vi "NXT_MIDBRAIN Wait For Buffer To Fill.vi"(4 "Buffer Length":u8, 5 "ModuleName":string, 6 "error in (no error)":errorcluster, 7 "Refnum in":T1) -> (2 "error out":errorcluster, 3 "Refnum out":T1)   [LabVIEW 2012]
uses:
  <vilib>/NXT/NXT Controls/NXTSyscallRefnum.ctl
  <resource>/objmgr/NXTInputOutput.rc
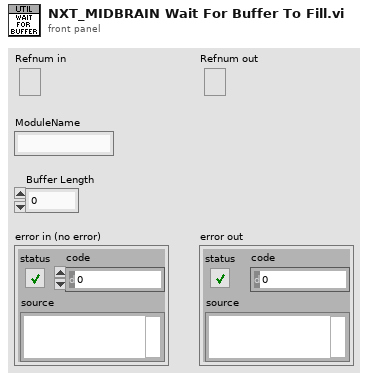
[diagram p1: front panel]
types:
  T1 = typedef "NXTSyscallRefnum.ctl" = refnum<k21>
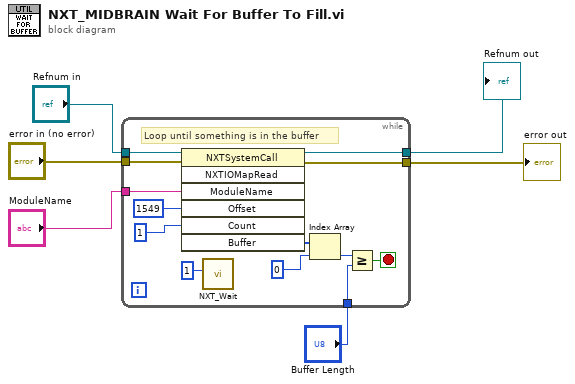
[diagram p0: block diagram]
diagram:
  n1 = while {
    tunnel: [w15] -> w3
    tunnel: [w14] -> w4
    tunnel: "Refnum in" -> [w13]
    tunnel: "error in (no error)" -> [w12]
    tunnel: "ModuleName" -> [w11]
    tunnel: "Buffer Length" -> [w7]
    stop <- w10 stop-if-true
    # "Loop until something is in the buffer"
    n2 = invoke class="NXTSystemCall" method="NXTIOMapRead"(reference=w13, error in=w12, "ModuleName"=w11, "Offset"=u16 1549, "Count"=u16 1) -> (reference out=w15:T1, error out=w14:errorcluster, "Buffer"=w18:u8[])  [unwired: 2 in, 4 out]
    n3 = call <vilib>:"NXT_Wait.vi"("Wait (ms)"=u32 1) -> ()  [unwired: 9 in, 2 out]
    n4 = Index Array(array=w18, index=0) -> (element=w8:u8)
    n5 = Greater Or Equal?(x=w8, y=w7) -> (x >= y?=w10:bool)
  }
  "error out" <- w4
  "Refnum out" <- w3
